vi "EOL All-Station Current Buffer.vi"(5 "Check sound?":bool, 7 "RS232 in":refnum<visa-resource-name>, 8 "Decibel data in":dbl[](array[numeric]), 9 "station idx":i32=4, 10 "Data Index In":i32, 11 "Data In":sgl[][](array[numeric])) -> (0 "Decibel data out":dbl[](array[numeric]), 2 "Data Index Out":i32, 3 "Data Out":sgl[][](array[numeric]))   [LabVIEW 2018]
panel:
  out "Waveform Graph":dbl[](graph)
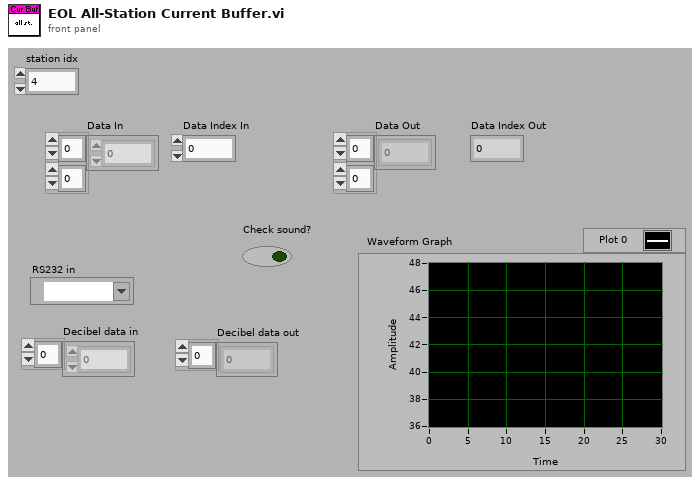
[diagram p1: front panel]
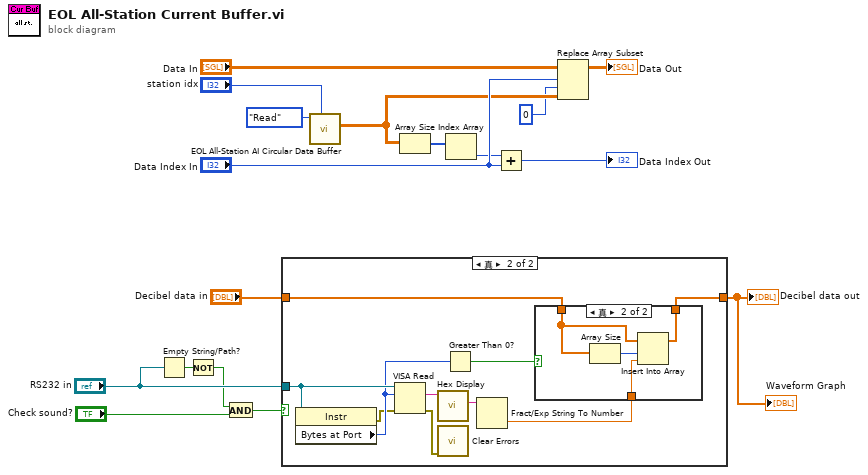
[diagram p0: block diagram]
diagram:
  n1 = Empty String/Path?(string/path="RS232 in") -> (empty?=w5:bool)
  n2 = Not(x=w5) -> (.not. x?=w4:bool)
  n3 = And(x=w4, y="Check sound?") -> (x .and. y?=w2:bool)
  n4 = case shown="真" w2 {
    tunnel: "RS232 in" -> [_ w28]
    tunnel: "Decibel data in" -> [w18 w26]
    tunnel: [w18 w27] -> w1
    frame False {
    }
    frame True {
      n5 = property class="Instr"(reference=w28) -> (error out=w19:errorcluster, "Bytes at Port"=w22:u32)  [unwired: 1 in, 1 out]
      n6 = VISA Read(VISA resource name=w28, byte count=w22, error in (no error)=w19) -> (read buffer=w24:string, error out=w20:errorcluster)  [unwired: 2 out]
      n7 = call "Hex Display.vi"("Hex Display"=w24) -> ("Display"=w23:string)  [unwired: 9 in, 1 out]
      n8 = call <vilib>:"Clear Errors.vi"("error in (no error)"=w20) -> ()  [unwired: 5 in, 2 out]
      n9 = Greater Than 0?(x=w22) -> (x > 0?=w21:bool)
      n10 = Fract/Exp String To Number(string=w23) -> (number=w25:dbl)  [unwired: 3 in, 1 out]
      n11 = case shown="真" w21 {
        tunnel: [w29 w32] -> w27
        tunnel: w26 -> [w29 w31]
        tunnel: w25 -> [_ w30]
        frame False {
        }
        frame True {
          n12 = Array Size(array=w31) -> (size(s)=w33:i32)
          n13 = Insert Into Array(array=w31, index=w33, new element=w30) -> (w32:dbl[])
        }
      }
    }
  }
  "Decibel data out" <- w1
  "Waveform Graph" <- w1
  n14 = call "EOL All-Station AI Circular Data Buffer.vi"("station idx"="station idx", "Mode"=enum16{"Initialize", "Read", "Write"}."Read") -> ("Data Read (Samp-Ro, Ch-Col)"=w10:sgl[][])  [unwired: 9 in]
  n15 = Array Size(array=w10) -> (size(s)=w13:i32[])
  n16 = Index Array(array=w13) -> (element=w9:i32)  [unwired: 1 in]
  n17 = Add(x=w9, y="Data Index In") -> (x+y=→"Data Index Out":i32)
  n18 = Replace Array Subset(array="Data In", new element=w10, index (row)="Data Index In", index (col)=0 ("disabled index (col)")) -> (→"Data Out":sgl[][])
